vi "niFpgaFFTStreamingStages_2048.vi"(0 "reset":bool, 1 "mult output type":fxp<+/-,18,2> format="%#.17g", 2 "bf bullet type":fxp<+/-,22,4>, 5 "bf data in":T1 {"x_r" format="%.16g"; "x_i" format="%.16g"; "y_r" format="%.16g"; "y_i" format="%.16g"}, 7 "stage switch in":bool, 9 "twiddle index in":fxp<+,10,10>, 11 "bf data type":T1 {"x_r" format="%.16g"; "x_i" format="%.16g"; "y_r" format="%.16g"; "y_i" format="%.16g"}) -> (6 "bf data out":T1 {"x_r" format="%.16g"; "x_i" format="%.16g"; "y_r" format="%.16g"; "y_i" format="%.16g"}, 8 "stage switch out":bool)   [LabVIEW 2017]
uses:
  <vilib>/rvi/Analysis/measure/FFT/supportingXNodes/permutation/templates/niFPGA FFT Perm Buffer 512 U32.vi
  <vilib>/rvi/Analysis/measure/FFT/supportingXNodes/BFGroup/templates/niFPGA BFGroup Input Buffer 2048 U32.vi
  <vilib>/rvi/Analysis/measure/FFT/supportingXNodes/BFGroup/templates/niFPGA BFGroup Twiddle Table 1024 U32.vi
  <vilib>/rvi/Analysis/measure/FFT/supportingXNodes/permutation/templates/niFPGA FFT Perm Buffer 128 U32.vi
  <vilib>/rvi/Analysis/measure/FFT/supportingXNodes/permutation/templates/niFPGA FFT Perm Buffer 256 U32.vi
  <vilib>/rvi/Analysis/measure/FFT/supportingXNodes/BFGroup/templates/niFPGA BFGroup Twiddle Table 256 U32.vi
  <vilib>/rvi/Analysis/measure/FFT/supportingXNodes/permutation/templates/niFPGA FFT Perm Buffer 64 U32.vi
  <vilib>/rvi/Analysis/measure/FFT/supportingXNodes/BFGroup/templates/niFPGA BFGroup Twiddle Table 64 U32.vi
  <vilib>/rvi/Analysis/measure/FFT/supportingXNodes/BFGroup/templates/niFPGA BFGroup Twiddle Table 16 U32.vi
  <vilib>/rvi/Analysis/measure/FFT/supportingXNodes/BFGroup/templates/niFPGA BFGroup Twiddle Table 4 U32.vi
  <vilib>/rvi/Analysis/measure/FFT/supportingXNodes/BFGroup/XNode/niFpgaFFTBFGroup.xnode
  <vilib>/rvi/FXPMathLib/basic elements/FxpDiscreteDelay/XNode/nifxpmath_DiscreteDelay.xnode
  <vilib>/rvi/Analysis/measure/FFT/supportingXNodes/permutation/XNode/niFpgaFFTPermutation.xnode
  <vilib>/rvi/Analysis/measure/FFT/supportingXNodes/butterfly/XNode/niFpgaFFTDIFButterfly.xnode
  <vilib>/rvi/FXPMathLib/FxpMul/XNode/nifxpmath_Multiplier.xnode
  <vilib>/rvi/FXPMathLib/sim/FxpSim.dll
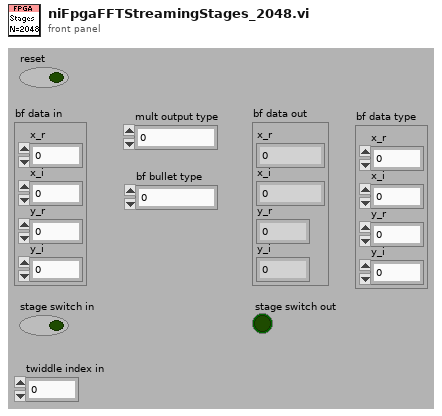
[diagram p1: front panel]
types:
  T1 = cluster{"x_r":fxp<+/-,16,1>, "x_i ":fxp<+/-,16,1>, "y_r ":fxp<+/-,16,1>, "y_i ":fxp<+/-,16,1>}
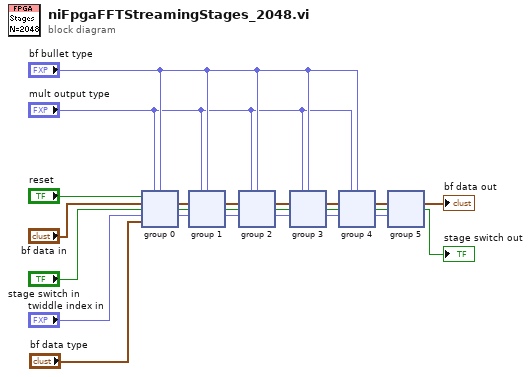
[diagram p0: block diagram]
diagram:
  n1 = xnode "group 0"("mult output type"="mult output type", "bf data in"="bf data in", "stage switch in"="stage switch in", "tf index in"="twiddle index in", "reset"="reset", "bf bullet type"="bf bullet type", "bf data type"="bf data type") -> ("stage switch out"=w23:bool, "bf data out"=w24:T1, "tf index out"=w22:fxp<+,10,10>)
  n2 = xnode "group 1"("mult output type"="mult output type", "bf data in"=w24, "stage switch in"=w23, "tf index in"=w22, "bf bullet type"="bf bullet type") -> ("stage switch out"=w20:bool, "bf data out"=w21:T1, "tf index out"=w19:fxp<+,10,10>)
  n3 = xnode "group 2"("mult output type"="mult output type", "bf data in"=w21, "stage switch in"=w20, "tf index in"=w19, "bf bullet type"="bf bullet type") -> ("stage switch out"=w17:bool, "bf data out"=w18:T1, "tf index out"=w16:fxp<+,10,10>)
  n4 = xnode "group 3"("mult output type"="mult output type", "bf data in"=w18, "stage switch in"=w17, "tf index in"=w16, "bf bullet type"="bf bullet type") -> ("stage switch out"=w13:bool, "bf data out"=w15:T1, "tf index out"=w12:fxp<+,10,10>)
  n5 = xnode "group 4"("mult output type"="mult output type", "bf data in"=w15, "stage switch in"=w13, "tf index in"=w12, "bf bullet type"="bf bullet type") -> ("stage switch out"=w10:bool, "bf data out"=w14:T1, "tf index out"=w11:fxp<+,10,10>)
  n6 = xnode "group 5"("bf data in"=w14, "stage switch in"=w10, "tf index in"=w11) -> ("stage switch out"=→"stage switch out":bool, "bf data out"=→"bf data out":T1)
